vi "MGI Max & Min (by magnitude) DBL.vi"(2 "y":dbl, 3 "x":dbl) -> (0 "Closest to zero":dbl, 1 "Furthest from zero":dbl)   [LabVIEW 2016]
doc: "Sorts the two input values into which is furthest from zero (largest magnitude) and which is closest to zero (smallest magnitude). The signs of the inputs are preserved.\n\nFreeware from Moore Good Ideas, www.mooregoodideas.com. Do not remove this line."
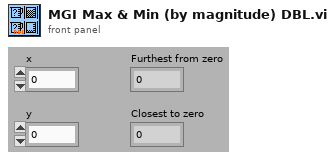
[diagram p1: front panel]
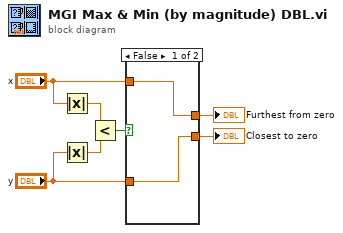
[diagram p0: block diagram]
diagram:
  n1 = Absolute Value(x="x") -> (abs(x)=w7:dbl)
  n2 = Absolute Value(x="y") -> (abs(x)=w6:dbl)
  n3 = Less?(x=w7, y=w6) -> (x < y?=w5:bool)
  n4 = case shown="False" w5 {
    tunnel: "x" -> [w9 w11]
    tunnel: "y" -> [w8 w10]
    tunnel: [w9 w10] -> w2
    tunnel: [w8 w11] -> w1
    frame False {
    }
    frame True {
    }
  }
  "Furthest from zero" <- w2
  "Closest to zero" <- w1
